vi "GetGP354Pressure.vi"() -> (3 "Pressure":dbl)   [LabVIEW 2011]
uses:
  GlobalVariables.vi
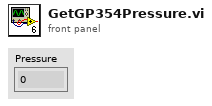
[diagram p1: front panel]
types:
  T1 = typedef "GP354 Cluster.ctl" = cluster{"Degas":bool, "Enable Filament 1":bool, "Enable Filament 2":bool, "Medium Emission":bool, "Ion Gauge":bool, "High Emission":bool, "Pressure":dbl}
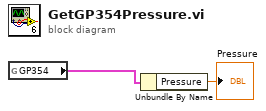
[diagram p0: block diagram]
diagram:
  n1 = global read "GlobalVariables.vi" "GP354"() -> (w1:T1)
  n2 = Unbundle By Name(w1) -> ("Pressure"=→"Pressure":dbl)
